vi "ExDataCollectFocusImageROT.vi"() -> ()   [LabVIEW 2016]
uses:
  Users/Public/Documents/SItoolkit/LabVIEW/ExamplesXX_6_0_2_9/Fast Examples/Open-Close Hardware/CamHandle.vi
panel:
  in  "Start wavelength":dbl=606.0
  in  "nm/pixel":dbl=0.101
  out "XY Graph":cluster{dbl[], dbl[]}(graph)
  out "Intensity Graph":sgl[][](graph)
  out "vert shift time":dbl format="%.2f"
  out "Read Out":dbl format="%.2f"
  in  "Stop collection":bool
  out "ready to \nstart":bool
  in  "Start collection":bool
  in  "Exposure":dbl=0.004 min=0.0 step=0.001 format="%.3f"
  out "error out":errorcluster
  in  "error in (no error)":errorcluster
  # "ExDataCollectImageROT:\nthis example collects data for Image.\nRun this vi and wait for the ready to start to turn green.\nThen hit the start button to collect and display the image in separate image display window.\nThis example will also display the readout time, horiztonal shift time, and the vertical shift time."
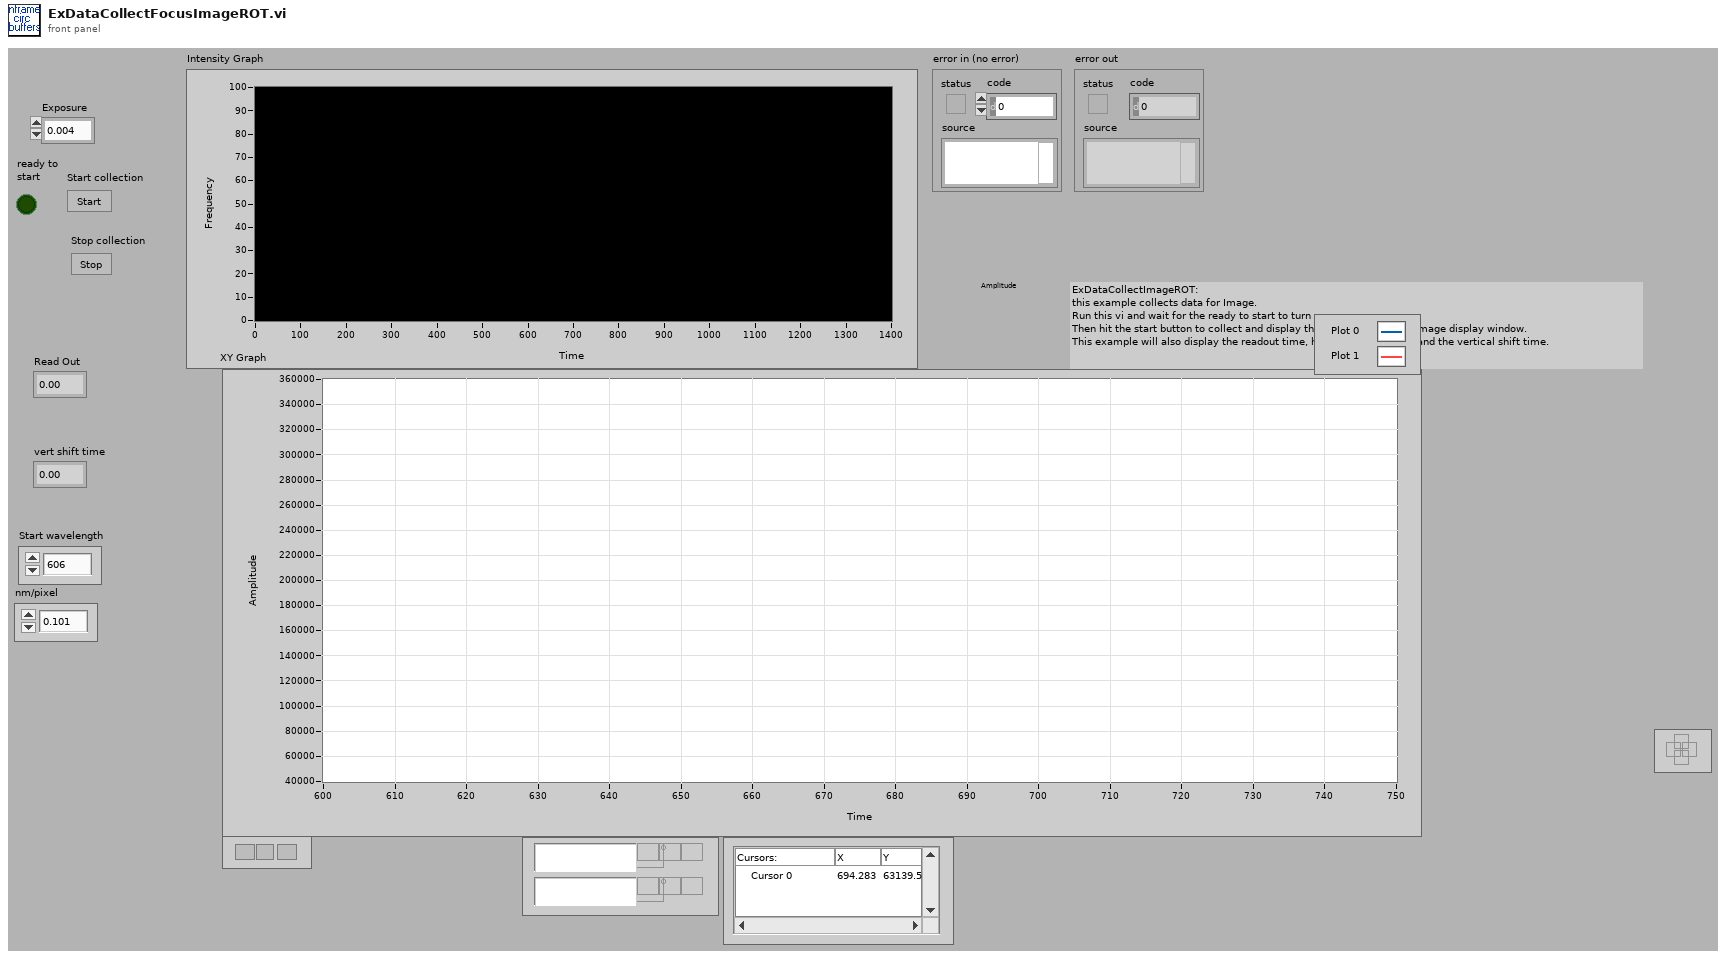
[diagram p1: front panel]
types:
  T1 = cluster{"acquire focus mode":u32, "Exposure":dbl, i32, "Software accumulation":u32}
  T2 = cluster{"Camera Handle":u32, "Pulser Handle":u32, "File Handle":u32, "Display Handle":u32, "Image Handle":u32}
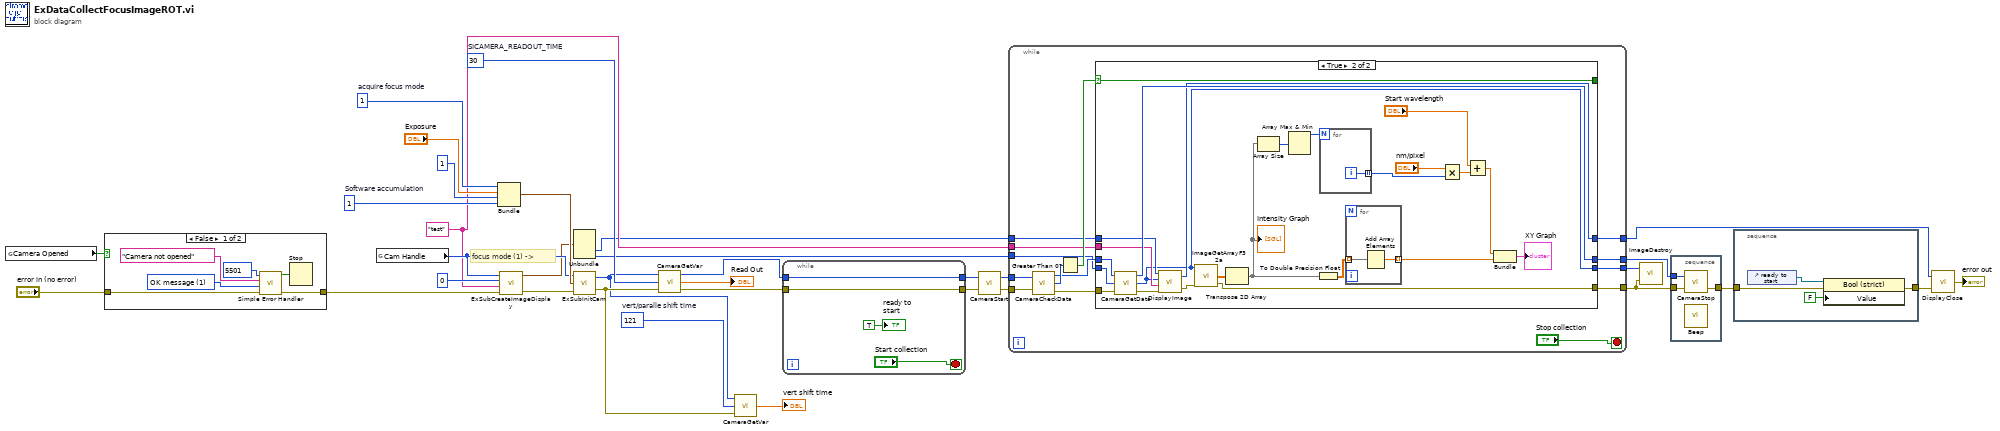
[diagram p0: block diagram]
diagram:
  w6 = "test"
  w12 = 121  # vert/paralle shift time
  w16 = 30  # SICAMERA_READOUT_TIME
  w32 = u32 1  # acquire focus mode
  w31 = u32 1  # Software accumulation
  # "focus mode (1) ->"
  n1 = global read "CamHandle.vi" "Camera Opened"() -> (w29:bool)
  n2 = case shown="False" w29 {
    tunnel: "error in (no error)" -> [w39 w41]
    tunnel: [w38 w41] -> w24
    frame False {
      w40 = u16 1 items=["no dialog", "OK message", "continue or stop message"] ("type of dialog (OK msg:1)")
      n3 = call <vilib>:"Simple Error Handler.vi"("error code (no error:0)"=5501, "error source (\" \")"="Camera not opened", "type of dialog (OK msg:1)"=w40, "error in (no error)"=w39) -> ("error?"=w36:bool, "error out"=w38:errorcluster)  [unwired: 1 in, 3 out]
      n4 = Stop(stop? (T)=w36) -> ()
    }
    frame True {
    }
  }
  n5 = global read "CamHandle.vi" "Cam Handle"() -> (w10:u32)
  n6 = Bundle("acquire focus mode"=w32, "Exposure"="Exposure", 1, "Software accumulation"=w31) -> (w33:T1)  [unwired: 1 in]
  n7 = call "ExSubCreateImageDisplay.vi"("Camera Handle"=w10, "Pulser Handle"=0, "File and Display Name"=w6, "error in (no error)"=w24) -> ("Handles Out"=w8:T2, "error out"=w23:errorcluster)  [unwired: 2 in]
  n8 = Unbundle(w8) -> ("Display Handle"=w5:u32, "Image Handle"=w7:u32)  [unwired: 3 out]
  n9 = call "ExSubInitCam.vi"("error in (no error)"=w23, "Camera Information"=w33, "Camera Handle"=w10) -> ("error out"=w15:errorcluster, "Camera Handle"=w13:u32)
  n10 = call <userlib>:"CameraGetVar.vi"("error in"=w15, "Parameter ID"=w16, "Camera Handle"=w13) -> ("error out"=w19:errorcluster, "Value"=→"Read Out":dbl, "Camera Handle"=w18:u32)
  n11 = call <userlib>:"CameraGetVar.vi"("error in"=w15, "Parameter ID"=w12, "Camera Handle"=w13) -> ("Value"=→"vert shift time":dbl)  [unwired: 2 out]
  n12 = while {
    tunnel: w19 -> [w43]
    tunnel: [w43] -> w28
    tunnel: w18 -> [w42]
    tunnel: [w42] -> w27
    stop <- "Start collection" stop-if-true
    "ready to \nstart" <- TRUE
  }
  n13 = call <userlib>:"CameraStart.vi"("error in"=w28, "Camera Handle"=w27) -> ("error out"=w25:errorcluster, "Camera Handle"=w26:u32)
  n14 = while {
    tunnel: w26 -> [w55]
    tunnel: w25 -> [w54]
    tunnel: [w52] -> w20
    tunnel: [w51] -> w22
    tunnel: w7 -> [w46]
    tunnel: w6 -> [w50]
    tunnel: w5 -> [w49]
    tunnel: [w48] -> w2
    tunnel: [w47] -> w1
    stop <- "Stop collection" stop-if-true
    n15 = call <userlib>:"CameraCheckData.vi"("Camera Handle"=w55, "error in"=w54) -> ("Camera Handle"=w57:u32, "Number Of Frames Available"=w59:i32, "error out"=w56:errorcluster)
    n16 = Greater Than 0?(x=w59) -> (x > 0?=w58:bool)
    n17 = case shown="True" w58 {
      selector: w58 -> [w63 w86]
      tunnel: w57 -> [w62 w88]
      tunnel: w56 -> [w64 w87]
      tunnel: [w63 w86] -> _
      tunnel: [w64 w78] -> w52
      tunnel: [w62 w85] -> w51
      tunnel: w50 -> [_ w82]
      tunnel: w49 -> [w61 w81]
      tunnel: [w61 w80] -> w48
      tunnel: [w60 w77] -> w47
      tunnel: w46 -> [w60 w84]
      frame False {
      }
      frame True {
        n18 = call <userlib>:"CameraGetData.vi"("error in"=w87, "Image/Data Handle"=w84, "Camera Handle"=w88) -> ("error out"=w83:errorcluster, "Image/Data Handle"=w77:u32, "Camera Handle"=w85:u32)
        n19 = call <userlib>:"DisplayImage.vi"("error in"=w83, "Title"=w82, "Image Handle"=w77, "Display Handle"=w81) -> ("error out"=w79:errorcluster, "Display Handle"=w80:u32)
        n20 = call <userlib>:"ImageGetArrayF32a.vi"("error in"=w79, "Data Handle"=w77) -> ("error out"=w78:errorcluster, "Array Float 32"=w76:sgl[][])  [unwired: 2 in, 1 out]
        n21 = Transpose 2D Array(2D array=w76) -> (transposed array=w65:sgl[][])
        "Intensity Graph" <- w65
        n22 = Array Size(array=w65) -> (size(s)=w75:i32[])
        n23 = Array Max & Min(array=w75) -> (max value=w73:i32)  [unwired: 3 out]
        n24 = To Double Precision Float(number=w65) -> (double precision float=w74:dbl[][])
        n25 = for {
          N: w73 -> [_]
          tunnel: [w91] -> w72 mode=indexing
          i -> [w91]
        }
        n26 = for {
          tunnel: w74 -> [w90] mode=indexing
          tunnel: [w89] -> w68 mode=indexing
          n27 = Add Array Elements(numeric array=w90) -> (sum=w89:dbl)
        }
        n28 = Multiply(x="nm/pixel", y=w72) -> (x*y=w71:dbl[])
        n29 = Add(x="Start wavelength", y=w71) -> (x+y=w70:dbl[])
        n30 = Bundle(w70, w68) -> (→"XY Graph":cluster{dbl[], dbl[]})  [unwired: 1 in]
      }
    }
  }
  n31 = call <userlib>:"ImageDestroy.vi"("error in"=w20, "Data handle"=w1) -> ()  [unwired: 1 out]
  n32 = stacked-sequence {
    tunnel: w22 -> [w94]
    tunnel: [w93] -> w21
    tunnel: w20 -> [w92]
    frame #0 {
      n33 = call <userlib>:"CameraStop.vi"("error in"=w92, "Camera Handle"=w94) -> ("error out"=w93:errorcluster)  [unwired: 1 out]
      n34 = call <vilib>:"Beep.vi"() -> ()  [unwired: 12 in]
    }
  }
  n35 = stacked-sequence {
    tunnel: [w96] -> w4
    tunnel: w21 -> [w95]
    frame #0 {
      n36 = control-ref of="ready to \nstart"() -> (w98:refnum<vi>)
      n37 = property class="Bool (strict)"(reference=w98, error in=w95, "Value"=FALSE) -> (error out=w96:errorcluster)  [unwired: 1 out]
    }
  }
  n38 = call <userlib>:"DisplayClose.vi"("error in"=w4, "Display Handle"=w2) -> ("error out"=→"error out":errorcluster)
